vi "Wait+.vi"(4 "Error In":errorcluster {"code" format="%.0x"}, 7 "milliseconds to wait":u32) -> (0 "Error Out":errorcluster {"code" format="%.0x"}, 3 "millisecond timer value":u32)   [LabVIEW 2018]
doc: "This VI is a simple wait in milliseconds with error clusters to use data flow techniques. It was obviously missing from the standard labVIEW distribution.\nScott Hannahs, <sth@magnet.fsu.edu> NHMFL-FSU, May 2003"
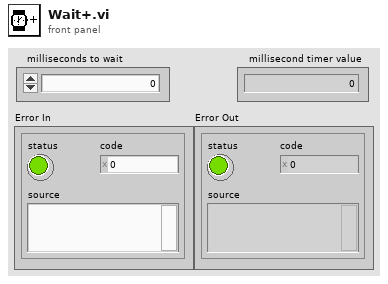
[diagram p1: front panel]
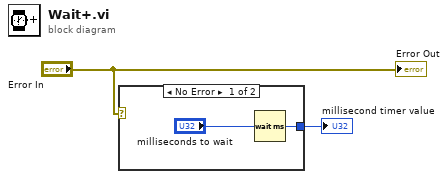
[diagram p0: block diagram]
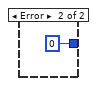
[diagram p2: hidden frame]
diagram:
  n1 = case shown="No Error" "Error In" {
    tunnel: [w3 u32 0 ("millisecond timer value")] -> w1
    frame No Error {
      n2 = Wait (ms)(milliseconds to wait="milliseconds to wait") -> (millisecond timer value=w3:u32)
    }
    frame Error {
    }
  }
  "millisecond timer value" <- w1
  "Error Out" <- "Error In"
